vi "GE 5565PIORC.DMA.Interrupt.Enable.vi"(8 "error in (no error)":errorcluster, 10 "enable (T)":bool=TRUE, 11 "GE 5565PIORC in":refnum<class "GE 5565PIORC.lvclass">) -> (0 "error out":errorcluster, 3 "GE 5565PIORC out":refnum<class "GE 5565PIORC.lvclass">)   [LabVIEW 2016, in "GE 5565PIORC.lvclass"]
doc: "Enables DMA interrupts for the provided GE 5565PIORC. When a DMA is completed, the GE 5565PIORC will generate an interrupt to the Host."
uses:
  GE 5565PIORC.lvclass
  GE 5565PIORC.lvclass/GE 5565PIORC.ctl
  Properties/Registers/GE 5565PIORC.Registers.Local Configuration.Read.vi
  Properties/Registers/GE 5565PIORC.Registers.Local Configuration.Read (U32).vi
  Properties/Registers/GE 5565PIORC.Registers.Local Configuration.Write.vi
  Properties/Registers/GE 5565PIORC.Registers.Local Configuration.Write (U32).vi
  GE 5565PIORC.Bit Manipulation.Set Bit.vi
  GE 5565PIORC.Bit Manipulation.Set Bit (U32).vi
  GE 5565PIORC.Registers.Read.vi
  GE 5565PIORC.Registers.Read (U32).vi
  GE 5565PIORC.Registers.Write.vi
  GE 5565PIORC.Registers.Write (U32).vi
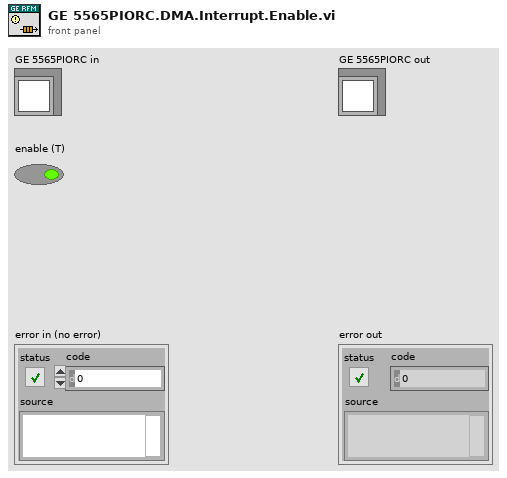
[diagram p1: front panel]
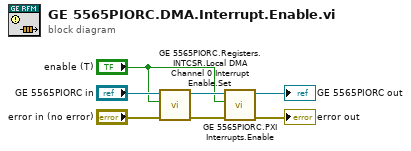
[diagram p0: block diagram]
diagram:
  n1 = call "GE 5565PIORC.Registers.INTCSR.Local DMA Channel 0 Interrupt Enable.Set.vi"("error in (no error)"="error in (no error)", "Local DMA Channel 0 Interrupt Enable"="enable (T)", "GE 5565PIORC in"="GE 5565PIORC in") -> ("error out"=w4:errorcluster, "GE 5565PIORC out"=w5:refnum<class "GE 5565PIORC.lvclass">)  [unwired: 7 in]
  n2 = call "GE 5565PIORC.PXI Interrupts.Enable.vi"("error in (no error)"=w4, "enable (T)"="enable (T)", "GE 5565PIORC in"=w5) -> ("error out"=→"error out":errorcluster, "GE 5565PIORC out"=→"GE 5565PIORC out":refnum<class "GE 5565PIORC.lvclass">)  [unwired: 7 in]
